vi "Init Msg Default.vi"() -> (2 "Msg":refnum<class "Msg.lvclass">)   [LabVIEW 2020, in "jettl.lvlib" / "Stopped jettl Msg.lvlib" / "Stopped.lvlib"]
uses:
  Stopped.lvlib
  Msg/Msg.lvclass
  Stopped Msg/Stopped Msg/Stopped Msg.lvclass
  Stopped Msg/Stopped Msg.lvlib
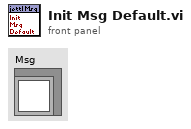
[diagram p1: front panel]
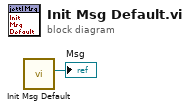
[diagram p0: block diagram]
diagram:
  n1 = call "Init Msg Default.vi"() -> ("Msg"=→"Msg":refnum<class "Msg.lvclass">)  [unwired: 11 in]
